vi "host.vi"() -> ()   [LabVIEW 2020]
uses:
  <vilib>/rvi/interface/RandomDataEmulation/nirviRandomDataOpen.vi
  <vilib>/rvi/interface/common/niFpgaCacheSessionInfoDynamic.vi
  <vilib>/Utility/error.llb/Error Cluster From Error Code.vi
  <vilib>/rvi/interface/common/niFpgaWaitOnOcc.vi
  <vilib>/rvi/errors/niLvFpgaAdjustHostInterfaceError.vi
  <vilib>/FPGAPlugInAG/Dynamic/niLvFpga_Run_Dynamic.vi
  <vilib>/FPGAPlugInAG/Dynamic/niLvFpga_Close_Dynamic.vi
  <vilib>/rvi/interface/nirviOpenFPGA/nirviOpenFPGA.xnode
  FFT.vi
  <vilib>/rvi/interface/nirviMethod/nirviMethod.xnode
  <vilib>/rvi/interface/nirviCloseFPGA/nirviCloseFPGA.xnode
  <vilib>/rvi/errors/niLvFpgaMergeErrorWithErrorCode.vi
  <vilib>/FPGAPlugInAG/Dynamic/niLvFpga_ReadFifo_Dynamic.vi
  <vilib>/Analysis/NI_AALPro.lvlib
  <vilib>/FPGAPlugInAG/Dynamic/niLvFpga_ConfigureFifo_Dynamic.vi
  <vilib>/FPGAPlugInAG/Dynamic/niLvFpga_StartFifo_Dynamic.vi
  <vilib>/FPGAPlugInAG/Dynamic/niLvFpga_WriteFifo_Dynamic.vi
panel:
  out "freq index":dbl[](array[numeric])
  out "truth/restored/final":dbl[][](graph)
  out "final signal trend add":dbl[](graph)
  out "restored   trend add":dbl[](graph)
  out "final signal":fxp<+/-,32,16>[](array[numeric])
  out "final signal":dbl[](graph)
  out "final signal":i32
  out "restored signal":dbl[](graph)
  out "restored signal size":i32
  out "restored signal":fxp<+/-,32,15>[](array[numeric])
  out "phase 2 index":dbl[](graph)
  out "phase 2 size":i32
  out "mag 2 index":dbl[](graph)
  out "mag 2 size":i32
  out "phase 2":fxp<+/-,32,15>[](array[numeric])
  out "mag 2":fxp<+/-,32,15>[](array[numeric])
  out "frequency index":dbl[](graph)
  out "frequency size":i32
  out "freq":fxp<+/-,32,15>[](array[numeric])
  out "magnitude":dbl[](graph)
  out "phase":dbl[](graph)
  out "phase size":i32
  out "mag size":i32
  out "phase":fxp<+/-,32,15>[](array[numeric])
  out "magnitude":fxp<+/-,32,15>[](array[numeric])
  out "Actual Depth":u32
  out "host to target":u32
  out "signal_target_to_host_fixed size(s)":i32
  out "target to host 1":u32
  out "signal target to host":dbl[][](graph)
  out "signal_target_to_host_fixed":fxp<+/-,24,7>[](array[numeric])
  out "Array 2":fxp<+/-,24,7>[](array[numeric])
  out "detrend acc":dbl[](graph)
  out "samples":i32
  out "input signal":T1(graph)
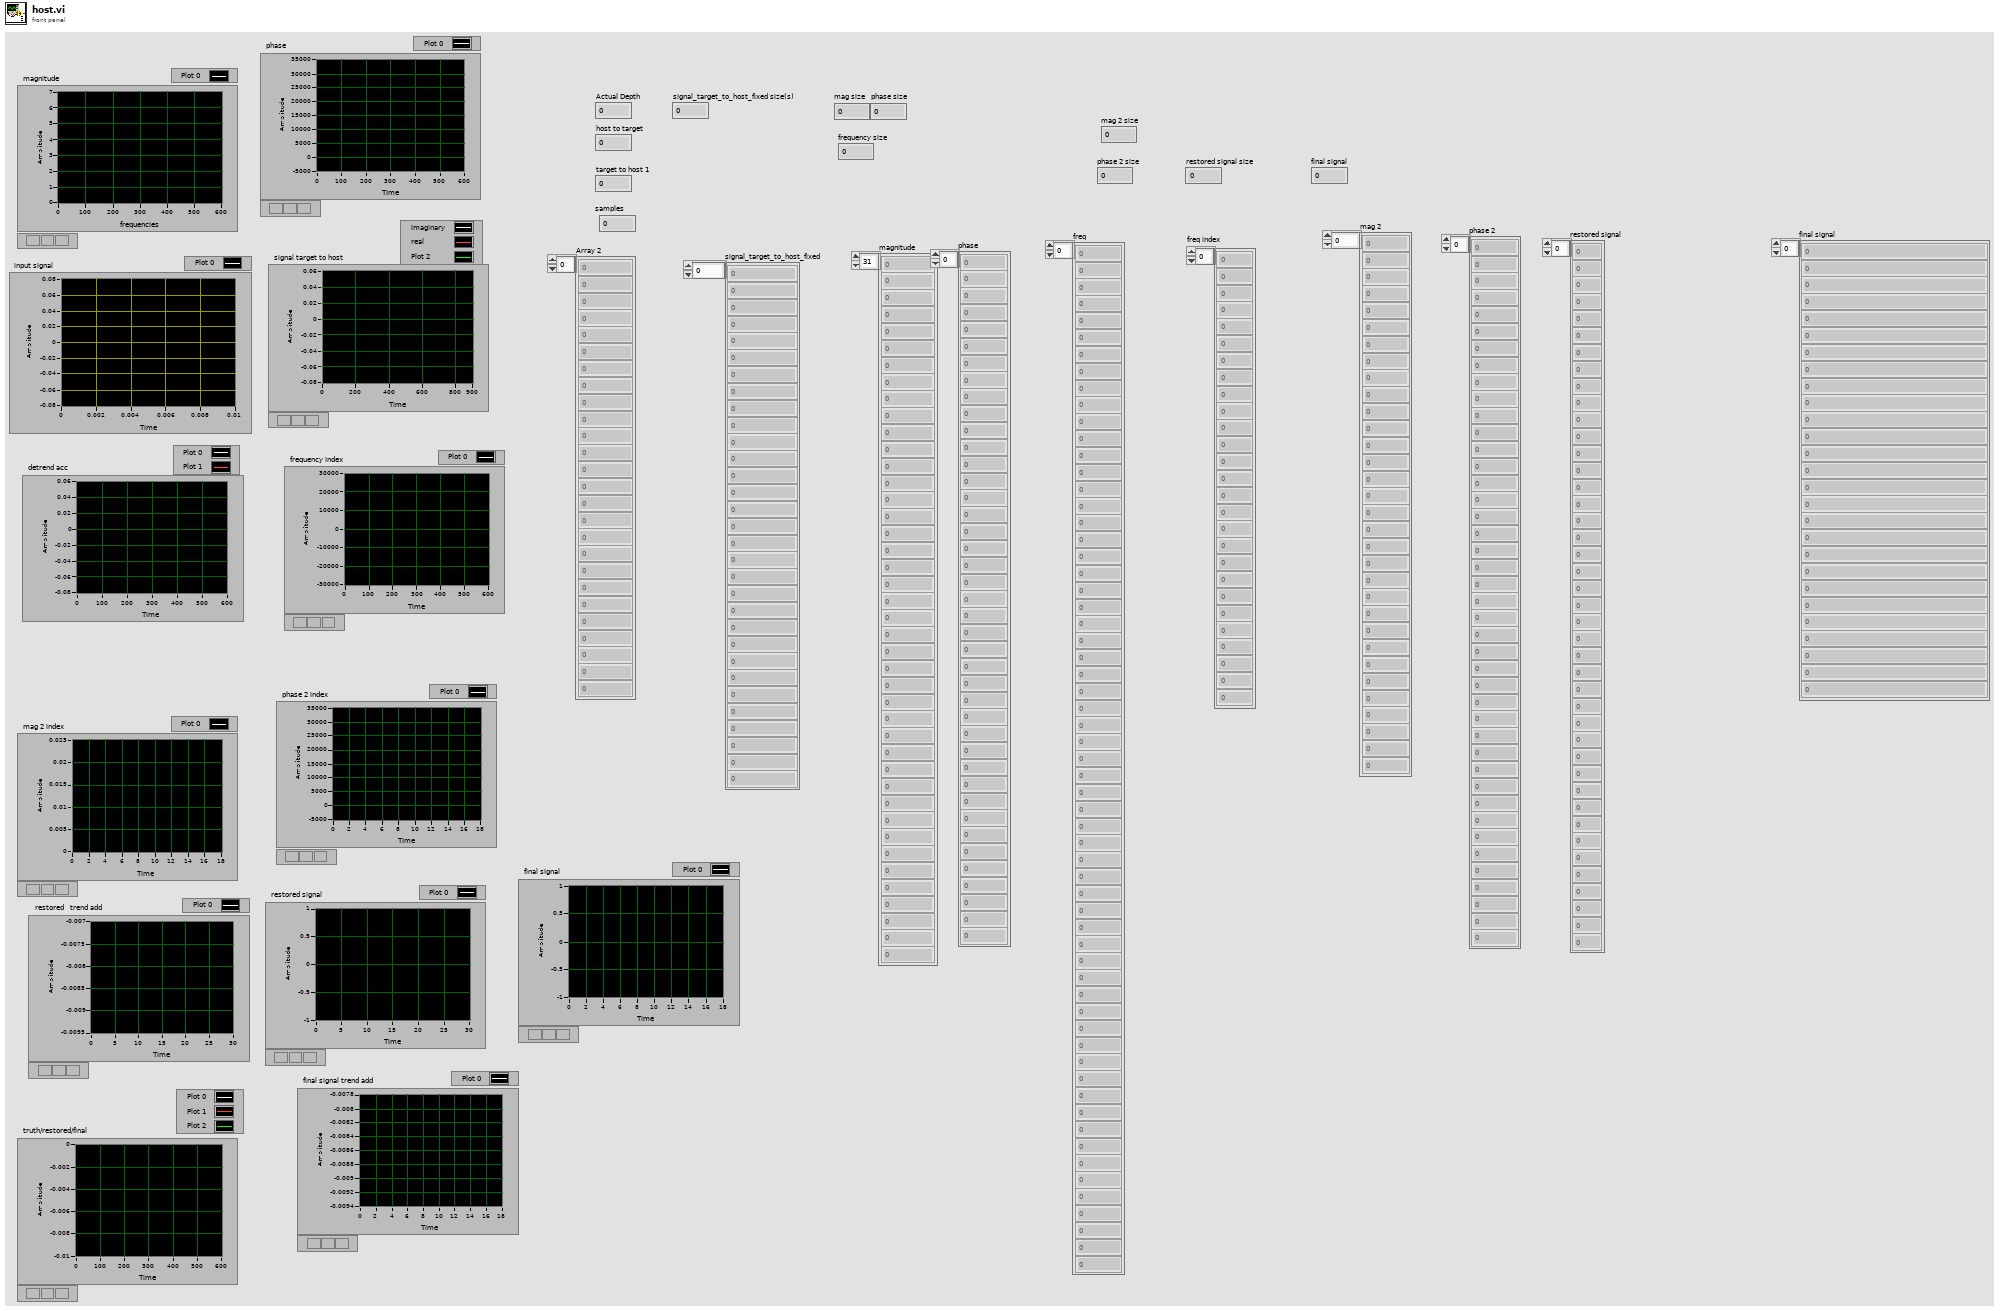
[diagram p1: front panel]
types:
  T1 = cluster{"array type (2D Dbl)":dbl[], "array type (2D Dbl)":dbl[]}
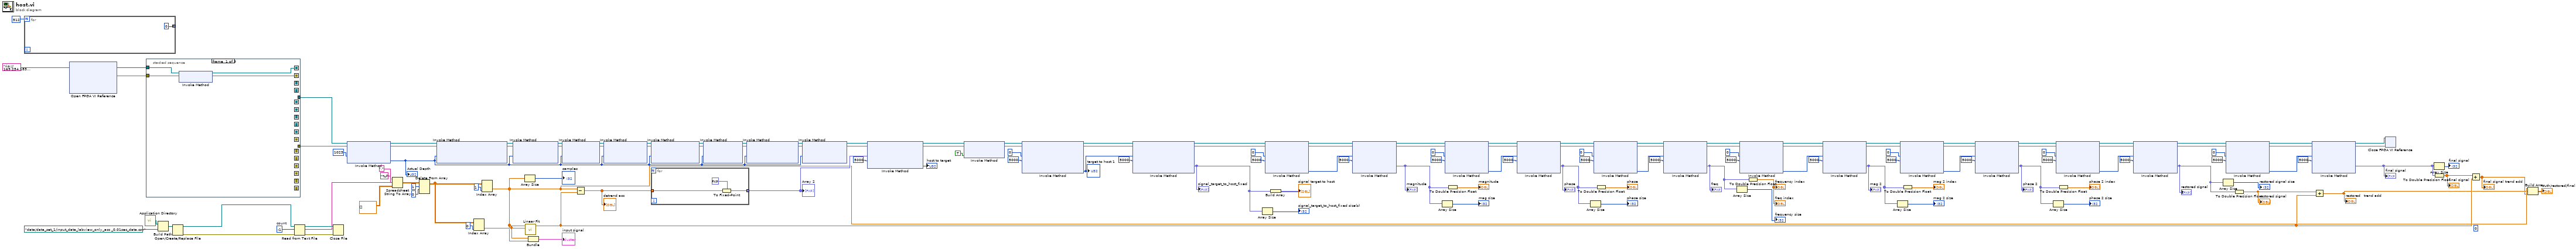
[diagram p0: block diagram]
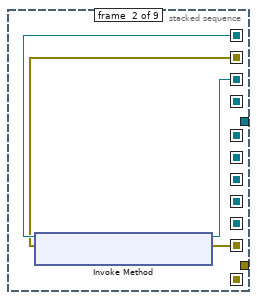
[diagram p2: hidden frame]
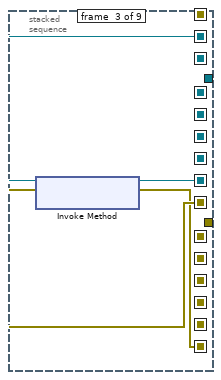
[diagram p3: hidden frame]
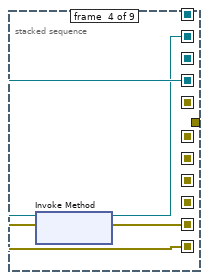
[diagram p4: hidden frame]
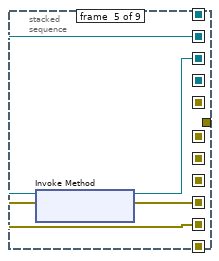
[diagram p5: hidden frame]
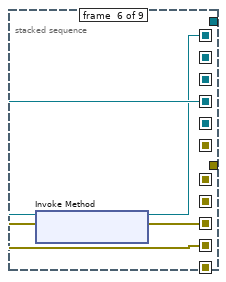
[diagram p6: hidden frame]
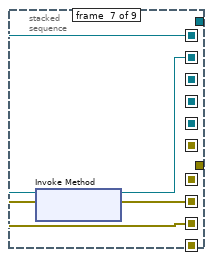
[diagram p7: hidden frame]
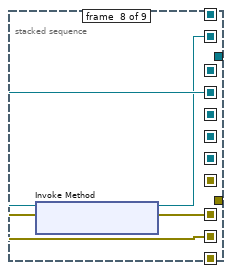
[diagram p8: hidden frame]
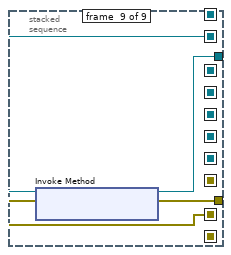
[diagram p9: hidden frame]
diagram:
  (unwired) 0 ("index")
  w140 = -1  # count
  n1 = for {
    N: 512 -> [_]
    tunnel: [0] -> _ mode=indexing
  }
  n2 = xnode "Open FPGA VI Reference"("resource name"=tag "rio://169.254.183.73/RIO0") -> ("FPGA VI Reference Out"=w110:refnum<k20>, "error out"=w109:errorcluster)  [unwired: 1 in]
  n3 = call <vilib>:"Application Directory.vi"() -> ("Application Directory"=w144:path)
  n4 = stacked-sequence {
    seq-local: [w152 _ _ _ _ _ _ _ _] -> [_ w158 _ _ _ _ _ _ _]
    seq-local: [w151 _ _ _ _ _ _ _ _] -> [_ w157 _ _ _ _ _ _ _]
    seq-local: [_ w156 _ _ _ _ _ _ _] -> [_ _ w162 _ _ _ _ _ _]
    seq-local: [_ w155 _ _ _ _ _ _ _] -> [_ _ w161 _ _ _ _ _ _]
    seq-local: [_ _ w160 _ _ _ _ _ _] -> [_ _ _ w166 _ _ _ _ _]
    seq-local: [_ _ w159 _ _ _ _ _ _] -> [_ _ _ w165 _ _ _ _ _]
    seq-local: [_ _ _ w164 _ _ _ _ _] -> [_ _ _ _ w170 _ _ _ _]
    seq-local: [_ _ _ w163 _ _ _ _ _] -> [_ _ _ _ w169 _ _ _ _]
    seq-local: [_ _ _ _ w168 _ _ _ _] -> [_ _ _ _ _ w174 _ _ _]
    seq-local: [_ _ _ _ w167 _ _ _ _] -> [_ _ _ _ _ w173 _ _ _]
    seq-local: [_ _ _ _ _ w172 _ _ _] -> [_ _ _ _ _ _ w178 _ _]
    seq-local: [_ _ _ _ _ w171 _ _ _] -> [_ _ _ _ _ _ w177 _ _]
    seq-local: [_ _ _ _ _ _ w176 _ _] -> [_ _ _ _ _ _ _ w181 _]
    seq-local: [_ _ _ _ _ _ w175 _ _] -> [_ _ _ _ _ _ _ w182 _]
    seq-local: [_ _ _ _ _ _ _ w180 _] -> [_ _ _ _ _ _ _ _ w186]
    seq-local: [_ _ _ _ _ _ _ w179 _] -> [_ _ _ _ _ _ _ _ w185]
    tunnel: w110 -> [w154 _ _ _ _ _ _ _ _]
    tunnel: w109 -> [w153 _ _ _ _ _ _ _ _]
    tunnel: [_ _ _ _ _ _ _ _ w184] -> w11
    tunnel: [_ _ _ _ _ _ _ _ w183] -> w10
    frame #0 {
      n5 = xnode "Invoke Method"("FPGA VI Reference In"=w154, "error in"=w153) -> ("FPGA VI Reference Out"=w152:refnum<k20>, "error out"=w151:errorcluster)
    }
    frame #1 {
      n6 = xnode "Invoke Method"("FPGA VI Reference In"=w158, "error in"=w157) -> ("FPGA VI Reference Out"=w156:refnum<k20>, "error out"=w155:errorcluster)
    }
    frame #2 {
      n7 = xnode "Invoke Method"("FPGA VI Reference In"=w162, "error in"=w161) -> ("FPGA VI Reference Out"=w160:refnum<k20>, "error out"=w159:errorcluster)
    }
    frame #3 {
      n8 = xnode "Invoke Method"("FPGA VI Reference In"=w166, "error in"=w165) -> ("FPGA VI Reference Out"=w164:refnum<k20>, "error out"=w163:errorcluster)
    }
    frame #4 {
      n9 = xnode "Invoke Method"("FPGA VI Reference In"=w170, "error in"=w169) -> ("FPGA VI Reference Out"=w168:refnum<k20>, "error out"=w167:errorcluster)
    }
    frame #5 {
      n10 = xnode "Invoke Method"("FPGA VI Reference In"=w174, "error in"=w173) -> ("FPGA VI Reference Out"=w172:refnum<k20>, "error out"=w171:errorcluster)
    }
    frame #6 {
      n11 = xnode "Invoke Method"("FPGA VI Reference In"=w178, "error in"=w177) -> ("FPGA VI Reference Out"=w175:refnum<k20>, "error out"=w176:errorcluster)
    }
    frame #7 {
      n12 = xnode "Invoke Method"("FPGA VI Reference In"=w182, "error in"=w181) -> ("FPGA VI Reference Out"=w180:refnum<k20>, "error out"=w179:errorcluster)
    }
    frame #8 {
      n13 = xnode "Invoke Method"("FPGA VI Reference In"=w186, "error in"=w185) -> ("FPGA VI Reference Out"=w184:refnum<k20>, "error out"=w183:errorcluster)
    }
  }
  n14 = Build Path(base path=w144, name or relative path=path "data/data_set_1/input_data_labview_only_acc _0.01sec_data.csv" ("default name")) -> (appended path=w143:path)
  n15 = Open/Create/Replace File(file path (use dialog)=w143) -> (refnum out=w148:refnum<file>, error out=w149:errorcluster)  [unwired: 5 in, 1 out]
  n16 = Read from Text File(file (use dialog)=w148, count=w140, error in=w149) -> (refnum out=w147:refnum<file>, text=w145:string, error out=w146:errorcluster)  [unwired: 1 in, 1 out]
  n17 = Close File(refnum=w147, error in=w146) -> ()  [unwired: 2 out]
  n18 = xnode "Invoke Method"("FPGA VI Reference In"=w11, "error in"=w10, "Requested Depth"=u32 1023) -> ("FPGA VI Reference Out"=w108:refnum<k20>, "error out"=w107:errorcluster, "Actual Depth"=w16:u32)
  "Actual Depth" <- w16
  n19 = Spreadsheet String To Array(delimiter (Tab)=",", format string="%f", spreadsheet string=w145, array type (2D Dbl)=dbl[][] []) -> (array=w137:dbl[][])
  n20 = Delete From Array(array=w137, length=1, index (row)=0) -> (array with subset deleted=w132:dbl[][])  [unwired: 1 in, 1 out]
  n21 = xnode "Invoke Method"("FPGA VI Reference In"=w108, "error in"=w107, "Requested Depth"=w16) -> ("FPGA VI Reference Out"=w106:refnum<k20>, "error out"=w105:errorcluster)  [unwired: 1 out]
  n22 = Index Array(array=w132, index (col)=0 ("disabled index (col)")) -> (element=w6:dbl[])  [unwired: 1 in]
  n23 = Index Array(array=w132, index (col)=1 ("disabled index (col)")) -> (element=w3:dbl[])  [unwired: 1 in]
  n24 = xnode "Invoke Method"("FPGA VI Reference In"=w106, "error in"=w105, "Requested Depth"=w16) -> ("FPGA VI Reference Out"=w104:refnum<k20>, "error out"=w103:errorcluster)  [unwired: 1 out]
  n25 = Array Size(array=w3) -> (size(s)=→"samples":i32)
  n26 = call <vilib>:"Linear Fit.vi"("Y"=w3, "X"=w6) -> ("Best Linear Fit"=w7:dbl[])  [unwired: 9 in, 4 out]
  n27 = Bundle("array type (2D Dbl)"=w6, "array type (2D Dbl)"=w3) -> (→"input signal":T1)  [unwired: 1 in]
  n28 = xnode "Invoke Method"("FPGA VI Reference In"=w104, "error in"=w103, "Requested Depth"=w16) -> ("FPGA VI Reference Out"=w70:refnum<k20>, "error out"=w69:errorcluster)  [unwired: 1 out]
  n29 = Subtract(x=w3, y=w7) -> (x-y=w124:dbl[])
  "detrend acc" <- w124
  n30 = xnode "Invoke Method"("FPGA VI Reference In"=w70, "error in"=w69, "Requested Depth"=w16) -> ("FPGA VI Reference Out"=w46:refnum<k20>, "error out"=w45:errorcluster)  [unwired: 1 out]
  n31 = xnode "Invoke Method"("FPGA VI Reference In"=w46, "error in"=w45, "Requested Depth"=w16) -> ("FPGA VI Reference Out"=w48:refnum<k20>, "error out"=w47:errorcluster)  [unwired: 1 out]
  n32 = for {
    tunnel: [w188] -> w123 mode=indexing
    tunnel: w124 -> [w187] mode=indexing
    n33 = To Fixed-Point(fixed-point type=fxp<+/-,24,7> 0.0 ("f"), number=w187) -> (fixed-point=w188:fxp<+/-,24,7>)
  }
  "Array 2" <- w123
  n34 = xnode "Invoke Method"("FPGA VI Reference In"=w48, "error in"=w47, "Requested Depth"=w16) -> ("FPGA VI Reference Out"=w31:refnum<k20>, "error out"=w30:errorcluster)  [unwired: 1 out]
  n35 = xnode "Invoke Method"("FPGA VI Reference In"=w31, "error in"=w30, "Requested Depth"=w16) -> ("FPGA VI Reference Out"=w15:refnum<k20>, "error out"=w14:errorcluster)  [unwired: 1 out]
  n36 = xnode "Invoke Method"("FPGA VI Reference In"=w15, "error in"=w14, "Requested Depth"=w16) -> ("FPGA VI Reference Out"=w13:refnum<k20>, "error out"=w12:errorcluster)  [unwired: 1 out]
  n37 = xnode "Invoke Method"("FPGA VI Reference In"=w13, "error in"=w12, "Data"=w123, "Timeout (ms)"=5000) -> ("FPGA VI Reference Out"=w129:refnum<k20>, "error out"=w128:errorcluster, "Empty Elements Remaining"=→"host to target":u32)
  n38 = xnode "Invoke Method"("FPGA VI Reference In"=w129, "error in"=w128, "Wait Until Done (F)"=TRUE) -> ("FPGA VI Reference Out"=w114:refnum<k20>, "error out"=w113:errorcluster)
  n39 = xnode "Invoke Method"("FPGA VI Reference In"=w114, "error in"=w113, "Number of Elements"=u32 0, "Timeout (ms)"=5000) -> ("FPGA VI Reference Out"=w122:refnum<k20>, "error out"=w121:errorcluster, "Elements Remaining"=w120:u32)  [unwired: 1 out]
  "target to host 1" <- w120
  n40 = xnode "Invoke Method"("FPGA VI Reference In"=w122, "error in"=w121, "Number of Elements"=w120, "Timeout (ms)"=5000) -> ("FPGA VI Reference Out"=w85:refnum<k20>, "error out"=w84:errorcluster, "Data"=w116:fxp<+/-,24,7>[])  [unwired: 1 out]
  "signal_target_to_host_fixed" <- w116
  n41 = Array Size(array=w116) -> (size(s)=→"signal_target_to_host_fixed size(s)":i32)
  n42 = xnode "Invoke Method"("FPGA VI Reference In"=w85, "error in"=w84, "Number of Elements"=u32 0, "Timeout (ms)"=5000) -> ("FPGA VI Reference Out"=w99:refnum<k20>, "error out"=w98:errorcluster, "Elements Remaining"=w93:u32)  [unwired: 1 out]
  n43 = Build Array(w116) -> (→"signal target to host":fxp<+/-,24,7>[][])
  n44 = xnode "Invoke Method"("FPGA VI Reference In"=w99, "error in"=w98, "Number of Elements"=w93, "Timeout (ms)"=5000) -> ("FPGA VI Reference Out"=w97:refnum<k20>, "error out"=w96:errorcluster, "Data"=w83:fxp<+/-,32,16>[])  [unwired: 1 out]
  "magnitude" <- w83
  n45 = Array Size(array=w83) -> (size(s)=→"mag size":i32)
  n46 = xnode "Invoke Method"("FPGA VI Reference In"=w97, "error in"=w96, "Number of Elements"=u32 0, "Timeout (ms)"=5000) -> ("FPGA VI Reference Out"=w95:refnum<k20>, "error out"=w94:errorcluster, "Elements Remaining"=w89:u32)  [unwired: 1 out]
  n47 = To Double Precision Float(number=w83) -> (double precision float=→"magnitude":dbl[])
  n48 = xnode "Invoke Method"("FPGA VI Reference In"=w95, "error in"=w94, "Number of Elements"=w89, "Timeout (ms)"=5000) -> ("FPGA VI Reference Out"=w72:refnum<k20>, "error out"=w71:errorcluster, "Data"=w82:fxp<+/-,32,16>[])  [unwired: 1 out]
  "phase" <- w82
  n49 = Array Size(array=w82) -> (size(s)=→"phase size":i32)
  n50 = xnode "Invoke Method"("FPGA VI Reference In"=w72, "error in"=w71, "Number of Elements"=u32 0, "Timeout (ms)"=5000) -> ("FPGA VI Reference Out"=w81:refnum<k20>, "error out"=w80:errorcluster, "Elements Remaining"=w77:u32)  [unwired: 1 out]
  n51 = To Double Precision Float(number=w82) -> (double precision float=→"phase":dbl[])
  n52 = xnode "Invoke Method"("FPGA VI Reference In"=w81, "error in"=w80, "Number of Elements"=w77, "Timeout (ms)"=5000) -> ("FPGA VI Reference Out"=w56:refnum<k20>, "error out"=w55:errorcluster, "Data"=w74:fxp<+/-,32,16>[])  [unwired: 1 out]
  "freq" <- w74
  n53 = Array Size(array=w74) -> (size(s)=→"frequency size":i32)
  n54 = xnode "Invoke Method"("FPGA VI Reference In"=w56, "error in"=w55, "Number of Elements"=u32 0, "Timeout (ms)"=5000) -> ("FPGA VI Reference Out"=w68:refnum<k20>, "error out"=w67:errorcluster, "Elements Remaining"=w64:u32)  [unwired: 1 out]
  n55 = To Double Precision Float(number=w74) -> (double precision float=→"frequency index" →"freq index":dbl[])
  n56 = xnode "Invoke Method"("FPGA VI Reference In"=w68, "error in"=w67, "Number of Elements"=w64, "Timeout (ms)"=5000) -> ("FPGA VI Reference Out"=w54:refnum<k20>, "error out"=w53:errorcluster, "Data"=w50:fxp<+/-,32,16>[])  [unwired: 1 out]
  "mag 2" <- w50
  n57 = Array Size(array=w50) -> (size(s)=→"mag 2 size":i32)
  n58 = xnode "Invoke Method"("FPGA VI Reference In"=w54, "error in"=w53, "Number of Elements"=u32 0, "Timeout (ms)"=5000) -> ("FPGA VI Reference Out"=w62:refnum<k20>, "error out"=w61:errorcluster, "Elements Remaining"=w58:u32)  [unwired: 1 out]
  n59 = To Double Precision Float(number=w50) -> (double precision float=→"mag 2 index":dbl[])
  n60 = xnode "Invoke Method"("FPGA VI Reference In"=w62, "error in"=w61, "Number of Elements"=w58, "Timeout (ms)"=5000) -> ("FPGA VI Reference Out"=w37:refnum<k20>, "error out"=w34:errorcluster, "Data"=w49:fxp<+/-,32,16>[])  [unwired: 1 out]
  "phase 2" <- w49
  n61 = Array Size(array=w49) -> (size(s)=→"phase 2 size":i32)
  n62 = xnode "Invoke Method"("FPGA VI Reference In"=w37, "error in"=w34, "Number of Elements"=u32 0, "Timeout (ms)"=5000) -> ("FPGA VI Reference Out"=w36:refnum<k20>, "error out"=w35:errorcluster, "Elements Remaining"=w39:u32)  [unwired: 1 out]
  n63 = To Double Precision Float(number=w49) -> (double precision float=→"phase 2 index":dbl[])
  n64 = xnode "Invoke Method"("FPGA VI Reference In"=w36, "error in"=w35, "Number of Elements"=w39, "Timeout (ms)"=5000) -> ("FPGA VI Reference Out"=w23:refnum<k20>, "error out"=w22:errorcluster, "Data"=w32:fxp<+/-,64,18>[])  [unwired: 1 out]
  "restored signal" <- w32
  n65 = Array Size(array=w32) -> (size(s)=→"restored signal size":i32)
  n66 = xnode "Invoke Method"("FPGA VI Reference In"=w23, "error in"=w22, "Number of Elements"=u32 0, "Timeout (ms)"=5000) -> ("FPGA VI Reference Out"=w26:refnum<k20>, "error out"=w25:errorcluster, "Elements Remaining"=w19:u32)  [unwired: 1 out]
  n67 = To Double Precision Float(number=w32) -> (double precision float=w9:dbl[])
  "restored signal" <- w9
  n68 = xnode "Invoke Method"("FPGA VI Reference In"=w26, "error in"=w25, "Number of Elements"=w19, "Timeout (ms)"=5000) -> ("FPGA VI Reference Out"=w21:refnum<k20>, "error out"=w20:errorcluster, "Data"=w17:fxp<+/-,32,16>[])  [unwired: 1 out]
  "final signal" <- w17
  n69 = Add(x=w9, y=w7) -> (x+y=w4:dbl[])
  "restored   trend add" <- w4
  n70 = xnode "Close FPGA VI Reference"("FPGA VI Reference In"=w21, "error in"=w20) -> ()  [unwired: 1 out]
  n71 = Array Size(array=w17) -> (size(s)=→"final signal":i32)
  n72 = To Double Precision Float(number=w17) -> (double precision float=w8:dbl[])
  "final signal" <- w8
  n73 = Add(x=w8, y=w7) -> (x+y=w1:dbl[])
  "final signal trend add" <- w1
  n74 = Build Array(w3, w4, w1) -> (→"truth/restored/final":dbl[][])
